vi "srv_data2tcpstr.vi"(10 "values":dbl[][](array[numeric]), 11 "tags":string) -> (3 "string array":string[](array[string]))   [LabVIEW 2013]
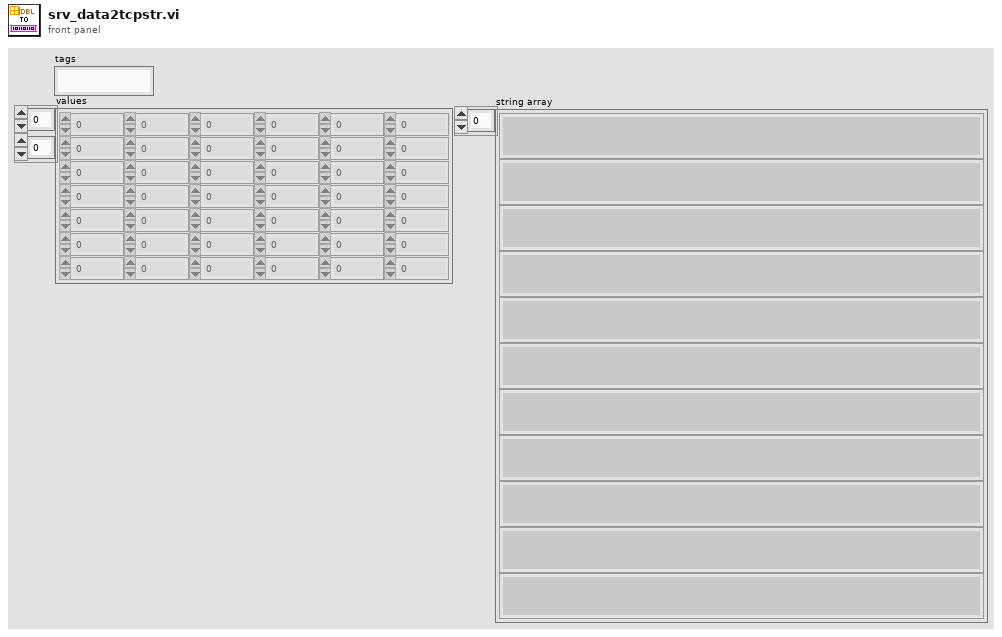
[diagram p1: front panel]
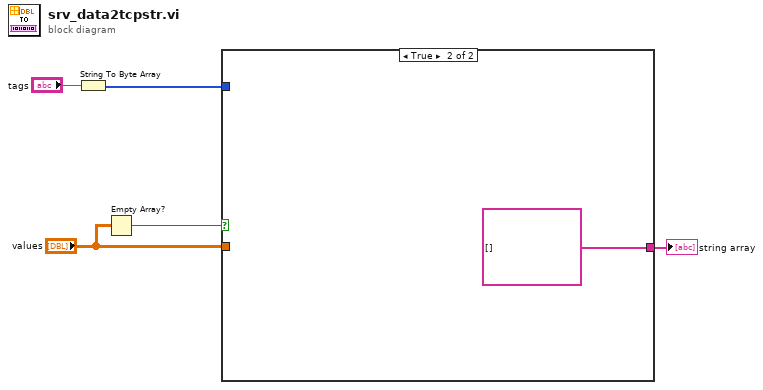
[diagram p0: block diagram]
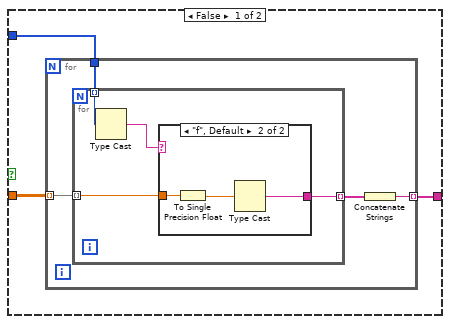
[diagram p2: hidden frame]
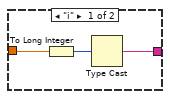
[diagram p3: hidden frame]
diagram:
  n1 = String To Byte Array(string="tags") -> (unsigned byte array=w4:u8[])
  n2 = Empty Array?(array="values") -> (empty?=w1:bool)
  n3 = case shown="True" w1 {
    tunnel: w4 -> [w8 _]
    tunnel: [w7 string[] []] -> w3
    tunnel: "values" -> [w6 _]
    frame False {
      n4 = for {
        tunnel: w6 -> [w12] mode=indexing
        tunnel: w8 -> [w11]
        tunnel: [w9] -> w7 mode=indexing
        n5 = for {
          tunnel: w12 -> [w14] mode=indexing
          tunnel: w11 -> [w16] mode=indexing
          tunnel: [w13] -> w10 mode=indexing
          n6 = Type Cast(x=w16) -> (*(type *) &x=w15:string)  [unwired: 1 in]
          n7 = case shown="\"f\", Default" w15 {
            tunnel: w14 -> [w17 w22]
            tunnel: [w18 w21] -> w13
            frame "i" {
              n8 = To Long Integer(number=w17) -> (32bit integer=w19:i32)
              n9 = Type Cast(x=w19) -> (*(type *) &x=w18:string)  [unwired: 1 in]
            }
            frame "f", Default {
              n10 = To Single Precision Float(number=w22) -> (single precision float=w20:sgl)
              n11 = Type Cast(x=w20) -> (*(type *) &x=w21:string)  [unwired: 1 in]
            }
          }
        }
        n12 = Concatenate Strings(w10) -> (w9:string)
      }
    }
    frame True {
    }
  }
  "string array" <- w3
